vi "Value Signaling Example.vi"() -> ()   [LabVIEW 2010]
panel:
  in  "Button 1":bool
  in  "Button 2":bool
  in  "Button 3":bool
  out "Event Structure\nTriggered":bool
  in  "stop":bool
  in  "Numeric Control":dbl
  # "Associated with a local variable.  Will not trigger the event structure."
  # "Manually changing this value\nwill trigger the event structure\nas it is a user event."
  # "Associated with a value property node.  Will not trigger the event structure."
  # "Associated with a signaling value\nproperty node.  This will trigger\nthe event structure."
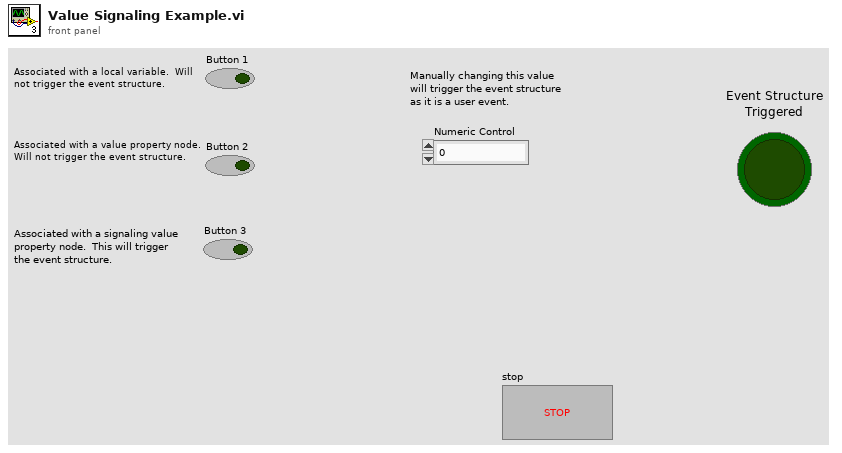
[diagram p1: front panel]
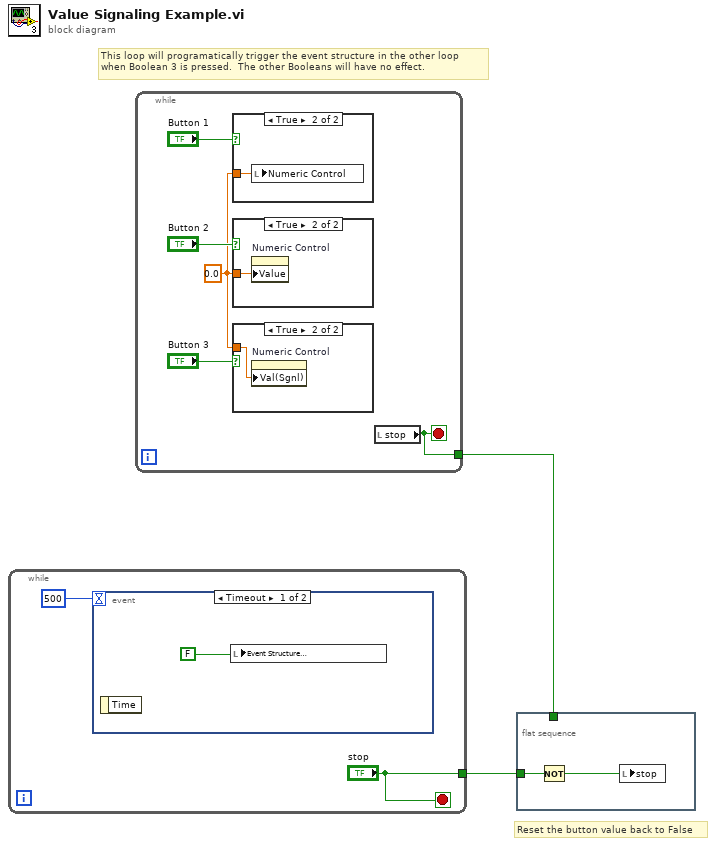
[diagram p0: block diagram]
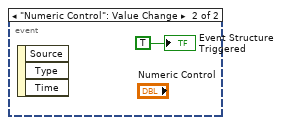
[diagram p2: hidden frame]
diagram:
  # "Reset the button value back to False"
  # "This loop will programatically trigger the event structure in the other loop\nwhen Boolean 3 is pressed.  The other Booleans will have no effect."
  n1 = while {
    tunnel: ["stop"] -> w2
    stop <- "stop" stop-if-true
    n2 = event shown="[0] Timeout" {
      selector: _ -> [_ _]
      dyn-events: _ -> [_ _]
      timeout: 500 -> [_ _]
      event Timeout {
        n3 = event-data() -> ()  [unwired: 1 in, 1 out]
        n4 = local write "Event Structure\nTriggered"(FALSE ("Boolean")) -> ()
      }
      event "Numeric Control": Value Change {
        n5 = event-data() -> ()  [unwired: 1 in, 3 out]
        "Event Structure\nTriggered" <- TRUE
      }
    }
  }
  n6 = while {
    tunnel: [w7] -> w1
    stop <- w7 stop-if-true
    w8 = 0.0
    n7 = case shown="True" "Button 1" {
      tunnel: w8 -> [_ w12]
      frame False {
      }
      frame True {
        n8 = local write "Numeric Control"(w12) -> ()
      }
    }
    n9 = case shown="True" "Button 2" {
      tunnel: w8 -> [_ w13]
      frame False {
      }
      frame True {
        n10 = property on="Numeric Control" class="DigNum (strict)"("Value"=w13) -> ()  [unwired: 2 in, 2 out]
      }
    }
    n11 = case shown="True" "Button 3" {
      tunnel: w8 -> [_ w14]
      frame False {
      }
      frame True {
        n12 = property on="Numeric Control" class="DigNum (strict)"("Val(Sgnl)"=w14) -> ()  [unwired: 2 in, 2 out]
      }
    }
    n13 = local read "stop"() -> (w7:bool)
  }
  n14 = flat-sequence {
    tunnel: w2 -> [w15]
    tunnel: w1 -> [_]
    frame #0 {
      n15 = Not(x=w15) -> (.not. x?=w16:bool)
      n16 = local write "stop"(w16) -> ()
    }
  }
